vi "Delete Queue.vi"(8 "error in (no error)":errorcluster, 10 "Queue":string, 11 "Azure Session in":refnum<class "Session.lvclass">) -> (0 "error out":errorcluster, 3 "Azure Session out":refnum<class "Session.lvclass">)   [LabVIEW 2015, in "NI_Azure_Queue.lvlib"]
doc: "Deletes a queue."
uses:
  NI_Azure_Queue.lvlib
  Core/Session/Session.lvclass
  Core/Session/Session.lvclass/Session.ctl
  Core/Session/Write HTTP Verb.vi
  Core/Session/Write URL Suffix.vi
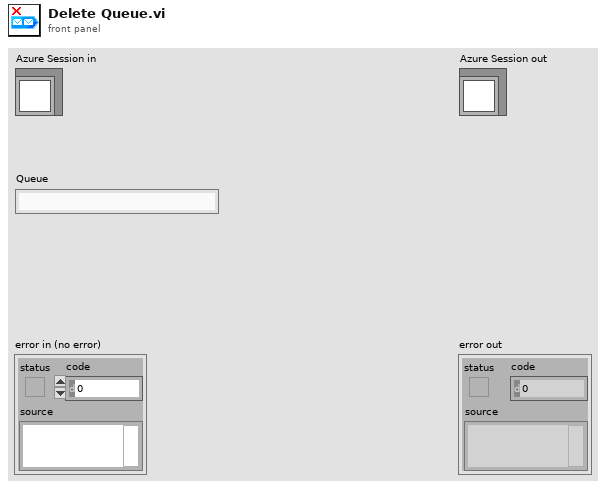
[diagram p1: front panel]
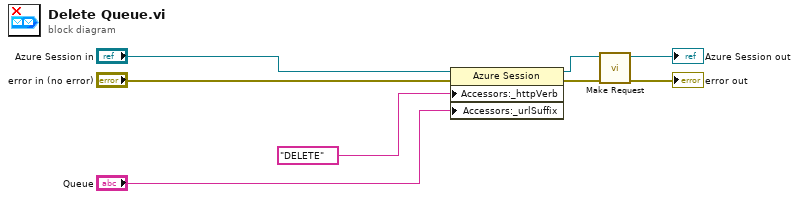
[diagram p0: block diagram]
diagram:
  n1 = property class="Azure Session"(reference="Azure Session in", error in="error in (no error)", "Accessors:_httpVerb"="DELETE" ("HTTP-Verb"), "Accessors:_urlSuffix"="Queue") -> (reference out=w3:refnum<class "Session.lvclass">, error out=w5:errorcluster)
  n2 = call "Make Request.vi"("error in (no error)"=w5, "Session in"=w3) -> ("error out"=→"error out":errorcluster, "Session out"=→"Azure Session out":refnum<class "Session.lvclass">)  [unwired: 7 in, 1 out]
